vi "动态显示.vi"(1 "停止按钮":bool, 2 "输入数据":string) -> (0 "暂存数据":string)   [LabVIEW 2015]
panel:
  out "动态显示数据":string
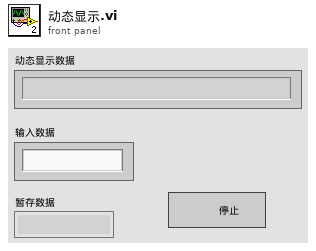
[diagram p1: front panel]
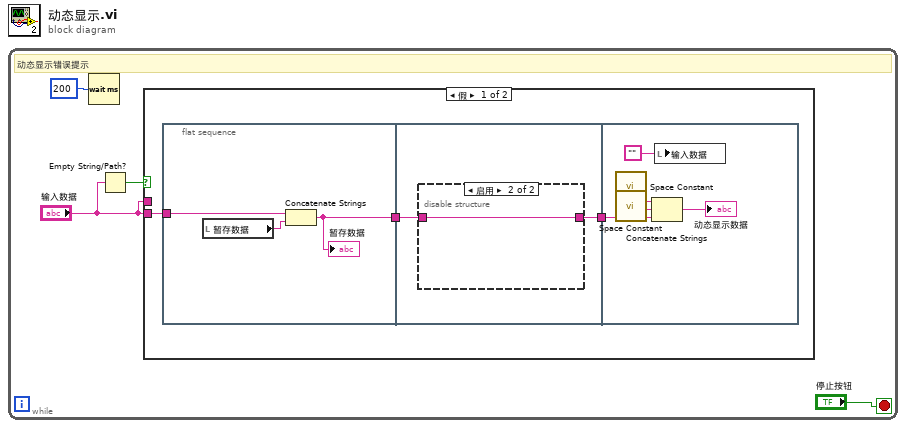
[diagram p0: block diagram]
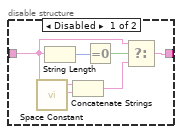
[diagram p2: hidden frame]
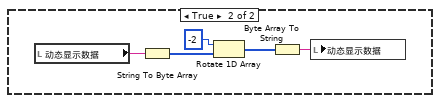
[diagram p3: hidden frame]
diagram:
  n1 = while {
    stop <- "停止按钮" stop-if-true
    # "动态显示错误提示"
    n2 = Wait (ms)(milliseconds to wait=u32 200 ("等待时间（毫秒）")) -> ()  [unwired: 1 out]
    n3 = Empty String/Path?(string/path="输入数据") -> (empty?=w3:bool)
    n4 = case shown="假" w3 {
      tunnel: "输入数据" -> [w7 _]
      tunnel: "输入数据" -> [_ _]
      frame False {
        n5 = flat-sequence {
          tunnel: w7 -> [w9]
          tunnel: [w10] -> w6
          tunnel: w6 -> [w11]
          tunnel: [w12] -> w5
          tunnel: w5 -> [w24]
          frame #0 {
            n6 = local read "暂存数据"() -> (w8:string)
            n7 = Concatenate Strings(w9, w8) -> (w10:string)
            "暂存数据" <- w10
          }
          frame #1 {
            n8 = disable-structure shown="启用" {
              disable-tunnel: [w16 w19] -> w12
              disable-tunnel: w11 -> [w15 w19]
              frame Disabled {
                n9 = call <vilib>:"Space Constant.vi"() -> ("String"=w13:string)
                n10 = String Length(string=w15) -> (length=w18:i32)
                n11 = Concatenate Strings(w15, w13) -> (w14:string)
                n12 = Equal To 0?(x=w18) -> (x = 0?=w17:bool)
                n13 = Select(t=w15, s=w17, f=w14) -> (s? t:f=w16:string)
              }
              frame Enabled {
              }
            }
          }
          frame #2 {
            n14 = call <vilib>:"Space Constant.vi"() -> ("String"=w22:string)
            n15 = call <vilib>:"Space Constant.vi"() -> ("String"=w23:string)
            n16 = Concatenate Strings(w22, w23, w24) -> (→"动态显示数据":string)
            n17 = local write "输入数据"("") -> ()
          }
        }
      }
      frame True {
        n18 = local read "动态显示数据"() -> (w25:string)
        n19 = String To Byte Array(string=w25) -> (unsigned byte array=w29:u8[])
        n20 = Rotate 1D Array(1:w29, 2:-2 ("n")) -> (0:w28:u8[])
        n21 = Byte Array To String(unsigned byte array=w28) -> (string=w26:string)
        n22 = local write "动态显示数据"(w26) -> ()
      }
    }
  }
